vi "Set Do.vi"(8 "error in (no error)":errorcluster, 9 "Indx":i32, 10 "Value":bool, 11 "FPGA_Concrete in":refnum<class "FPGA_Concrete.lvclass">) -> (0 "error out":errorcluster, 3 "FPGA_Concrete out":refnum<class "FPGA_Concrete.lvclass">)   [LabVIEW 2019, in "FPGA_Concrete.lvclass"]
uses:
  FPGA_Concrete.lvclass
  <vilib>/Utility/error.llb/Error Cluster From Error Code.vi
  <vilib>/ErrorRing/Error Ring.xnode
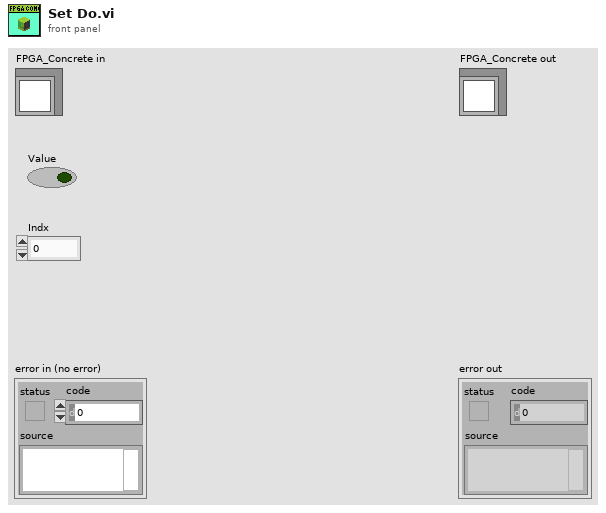
[diagram p1: front panel]
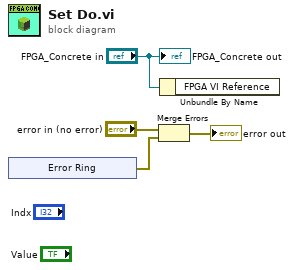
[diagram p0: block diagram]
diagram:
  n1 = xnode "Error Ring"() -> ("error out"=w2:errorcluster)
  n2 = Merge Errors("error in (no error)", w2) -> (→"error out":errorcluster)
  n3 = Unbundle By Name("FPGA_Concrete in") -> ()  [unwired: 1 out]
  "FPGA_Concrete out" <- "FPGA_Concrete in"
